vi "Vision - Get Initial Image Size.vi"(6 "Panel Size":T2, 8 "error in (no error)":errorcluster, 10 "Rectangle":T3, 11 "ThumbNail Dims in":T1) -> (0 "error out":errorcluster, 1 "Draw Area Size":T2)   [LabVIEW 2024]
uses:
  <vilib>/Utility/miscctls.llb/LVBoundsTypeDef.ctl
  Controls/ThumbNail Dimensions.ctl
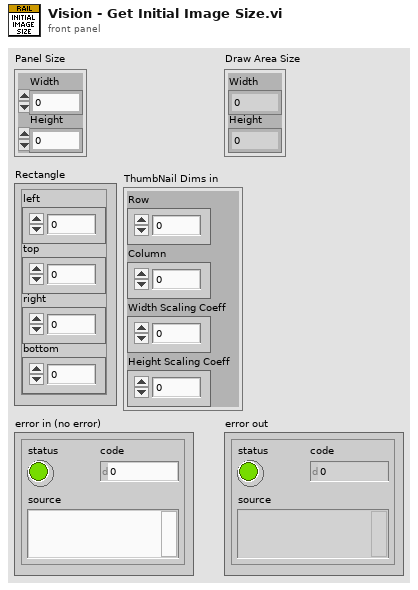
[diagram p1: front panel]
types:
  T1 = typedef "ThumbNail Dimensions.ctl" = cluster{"Row":i32, "Column":i32, "Width Scaling Coeff":dbl, "Height Scaling Coeff":dbl}
  T2 = typedef "LVBoundsTypeDef.ctl" = cluster{"Width":u32, "Height":u32}
  T3 = cluster{"left":i16, "top":i16, "right":i16, "bottom":i16}
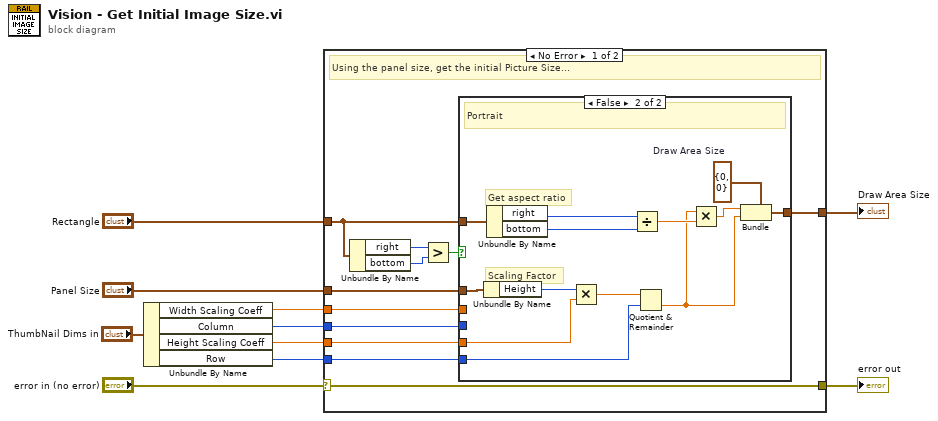
[diagram p0: block diagram]
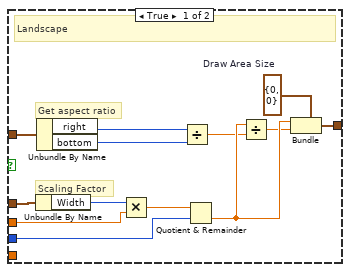
[diagram p2: hidden frame]
diagram:
  n1 = Unbundle By Name("ThumbNail Dims in") -> ("Width Scaling Coeff"=w4:dbl, "Column"=w3:i32, "Height Scaling Coeff"=w2:dbl, "Row"=w1:i32)
  n2 = case shown="No Error" "error in (no error)" {
    selector: "error in (no error)" -> [w18 w48]
    tunnel: [w21 _] -> w6
    tunnel: w4 -> [w20 _]
    tunnel: "Panel Size" -> [w17 _]
    tunnel: "Rectangle" -> [w13 _]
    tunnel: w3 -> [w19 _]
    tunnel: [w18 w48] -> w10
    tunnel: w2 -> [w12 _]
    tunnel: w1 -> [w11 _]
    frame No Error {
      # "Using the panel size, get the initial Picture Size..."
      n3 = Unbundle By Name(w13) -> ("right"=w16:i16, "bottom"=w15:i16)
      n4 = Greater?(x=w16, y=w15) -> (0:w14:bool)
      n5 = case shown="False" w14 {
        tunnel: [w26 w41] -> w21
        tunnel: w20 -> [w25 _]
        tunnel: w13 -> [w24 w40]
        tunnel: w19 -> [w23 _]
        tunnel: w17 -> [w22 w39]
        tunnel: w12 -> [_ w38]
        tunnel: w11 -> [_ w37]
        frame True {
          w31 = T2 {"Width"=0, "Height"=0}  # Draw Area Size
          # "Scaling Factor"
          # "Get aspect ratio"
          # "Landscape"
          n6 = Unbundle By Name(w22) -> ("Width"=w34:u32)
          n7 = Unbundle By Name(w24) -> ("right"=w33:i16, "bottom"=w32:i16)
          n8 = Multiply(x=w34, y=w25) -> (x*y=w30:dbl)
          n9 = Divide(x=w33, y=w32) -> (x/y=w28:dbl)
          n10 = Quotient & Remainder(x=w30, y=w23) -> (floor(x/y)=w29:dbl)  [unwired: 1 out]
          n11 = Divide(x=w29, y=w28) -> (x/y=w27:dbl)
          n12 = Bundle(cluster=w31, "Width"=w29, "Height"=w27) -> (w26:T2)
        }
        frame False {
          w44 = T2 {"Width"=0, "Height"=0}  # Draw Area Size
          # "Scaling Factor"
          # "Get aspect ratio"
          # "Portrait"
          n13 = Unbundle By Name(w39) -> ("Height"=w47:u32)
          n14 = Unbundle By Name(w40) -> ("right"=w46:i16, "bottom"=w45:i16)
          n15 = Multiply(x=w47, y=w38) -> (x*y=w43:dbl)
          n16 = Divide(x=w46, y=w45) -> (x/y=w42:dbl)
          n17 = Quotient & Remainder(x=w43, y=w37) -> (floor(x/y)=w35:dbl)  [unwired: 1 out]
          n18 = Multiply(x=w35, y=w42) -> (x*y=w36:dbl)
          n19 = Bundle(cluster=w44, "Width"=w36, "Height"=w35) -> (w41:T2)
        }
      }
    }
    frame Error {
    }
  }
  "error out" <- w10
  "Draw Area Size" <- w6
